vi "PID with autotuning.vi"(0 "gain scheduling variable":dbl format="%.2f", 4 "iteration":i32, 5 "autotuning parameters":T5={"Controller Type"=0, "# of cycles to avg"=3, "Relay amplitude"=2.0, "Control design  "=0, "Noise level"=0.1} {"Noise level" format="%.2f"; "Control design" items=["Normal", "Fast", "Slow"]; "Relay amplitude" format="%.2f"; "Controller Type" items=["PID", "PI", "P"]}, 6 "options":T3={"sp low"=0.0, "sp high"=100.0, "out low"=-100.0, "out high"=100.0, "hold (F)"=FALSE, "auto (T)"=TRUE, "pro. band (F)"=FALSE, "reverse acting (T)"=TRUE, "beta"=1.0, "linearity"=1.0, "dt (s)"=-1.0} {"dt (s)" format="%.2f"; "linearity" min=0.0 max=1.0 format="%.2f"; "sp low" format="%.2f"; "sp high" format="%.2f"; "out low" format="%.2f"; "out high" format="%.2f"; "beta" min=0.0 max=1.0 format="%.2f"}, 7 "autotune? (F)":bool, 8 "manual control":dbl(slide)=5.551115123125783e-15 scale=-100.0..100.0 scale format="%.1f", 9 "gain scheduling":T2={"gain schedule"=[100.0], "PID parameters"=[{"Kc"=4.851751673610237, "Ti (min)"=0.021111111111111112, "Td (min)"=0.005277777777777778}], "scheduling input"=0} {"scheduling input" items=["Setpoint", "Process variable", "Controller output", "Gain scheduling input"]; "PID parameters"."Td (min)" format="%.4f"; "PID parameters"."Ti (min)" format="%.4f"; "PID parameters"."Kc" format="%.4f"; "gain schedule" format="%.2f"}, 10 "process variable":dbl(slide)=29.68036460876465 scale=0.0..100.0 scale format="%.1f", 11 "setpoint":dbl(slide)=30.35714340209961 scale=0.0..100.0 scale format="%.1f") -> (1 "updated parameters":T2={"gain schedule"=[100.0], "PID parameters"=[{"Kc"=4.851751673610237, "Ti (min)"=0.021111111111111112, "Td (min)"=0.005277777777777778}], "scheduling input"=0} {"scheduling input" items=["Setpoint", "Process variable", "Controller output", "Gain scheduling input"]; "PID parameters"."Td (min)" format="%.4f"; "PID parameters"."Ti (min)" format="%.4f"; "PID parameters"."Kc" format="%.4f"; "gain schedule" format="%.2f"}, 2 "tuning completed?":bool, 3 "output":dbl(slide)=-0.9174311757087708 scale=-100.0..100.0 scale format="%.1f")   [LabVIEW 2020, in "NI_PID__autopid compat.lvlib"]
doc: "This VI can be used as a basic PID VI with gain scheduling. In addition, the VI has inputs used to specify and initiate a setpoint relay autotuning procedure. Passing a TRUE value to the autotune? input initiates the autotuning wizard.\n\nDescription of the PID algorithm:\n\nDerivative action is on the process variable only. Anti-reset windup and bumpless transfer are supported.\n\nThis VI should be called from inside a while loop with a fixed cycle time. If Cycle Time is less than or equal to zero, an internal timer with 1 millisecond resolution is used for calculations.\n\nThis VI is reentrant, so you can call it from multiple, independent higher-level VIs without interference.\n\nThe default variable ranges correspond to setpoint, process variable, and output expressed in percent. Reverse action (also called increase-decrease) is the \"normal\" controller mode where the output decreases if the process variable is higher than the setpoint.\n\nSwitching from auto to manual is bumpless; the initial value of the Manual Output control is subtracted out so that it is really a \"relative\" output control. Switching from manual to auto is also bumpless.\n\nSwitching to Hold causes the controller to ignore further changes in the process variable and suspends any integral action. Thus, the output stays constant at the last value."
uses:
  <vilib>/addons/control/pid/NI_PID__autopid compat.lvlib
  <vilib>/addons/control/pid/NI_PID__prctrl compat.lvlib
panel:
  in  "Dummy":T1 {"Td" format="%.2f"; "Ti" format="%.2f"; "Kc" format="%.2f"}
  in  "states":T4(ring)=enum."Start"
  # "SP & PV range:"
  # "Output range:"
  # "-1: default,using\nsystem clock"
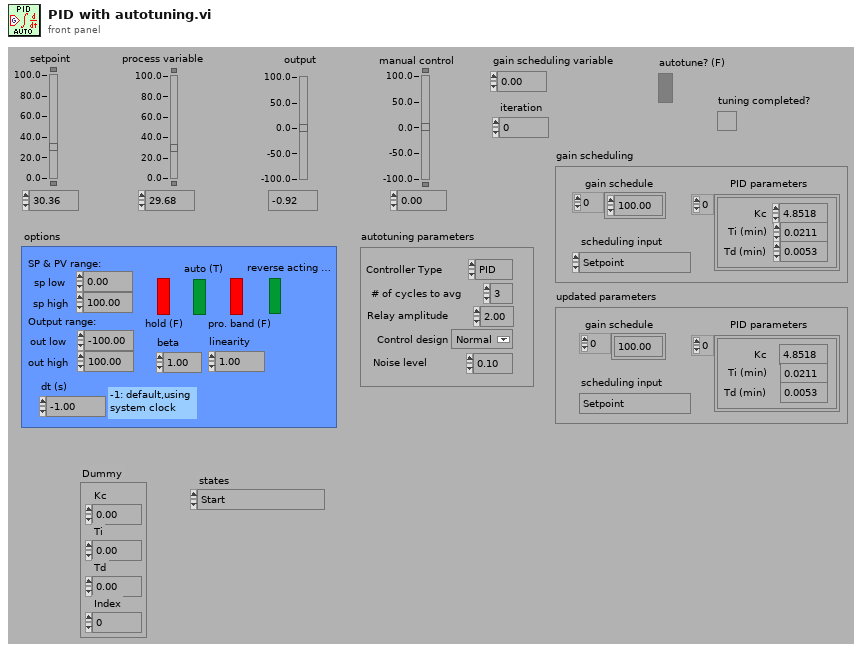
[diagram p1: front panel]
types:
  T1 = cluster{"Kc":dbl, "Ti":dbl, "Td":dbl, "Index":i32}
  T2 = cluster{"gain schedule":dbl[], "PID parameters":cluster{"Kc":dbl, "Ti (min)":dbl, "Td (min)":dbl}[], "scheduling input":u16}
  T3 = cluster{"sp low":dbl, "sp high":dbl, "out low":dbl, "out high":dbl, "hold (F)":bool, "auto (T)":bool, "pro. band (F)":bool, "reverse acting (T)":bool, "beta":dbl, "linearity":dbl, "dt (s)":dbl}
  T4 = enum16{"Normal", "Start", "Check params", "Check noise", "Start noise est.", "Re-estimate noise", "Begin autotune", "Autotuning", "New parameters", ""}
  T5 = cluster{"Controller Type":u16, "# of cycles to avg":i32, "Relay amplitude":dbl, "Control design  ":u16, "Noise level":dbl}
  T6 = cluster{"process variable":dbl, "setpoint relay":dbl, "output":dbl}
  T7 = cluster{"PB (%)":dbl, "Reset (min)":dbl, "Rate (min)":dbl, "Index":i32}
  T8 = cluster{"Kc":dbl, "Ti (min)":dbl, "Td (min)":dbl}[]
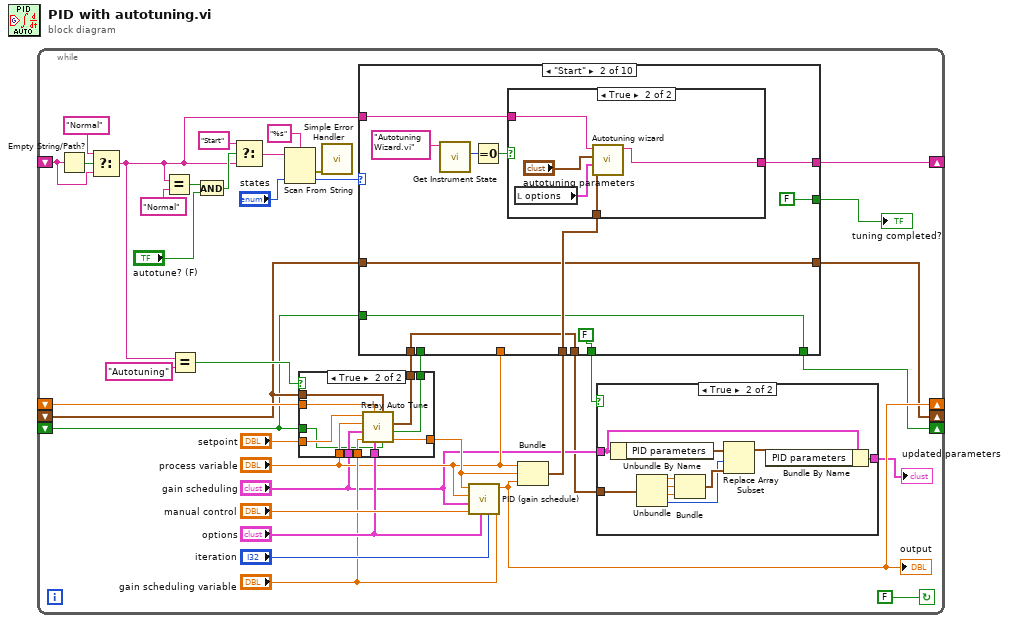
[diagram p0: block diagram]
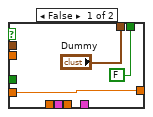
[diagram p3: hidden frame]
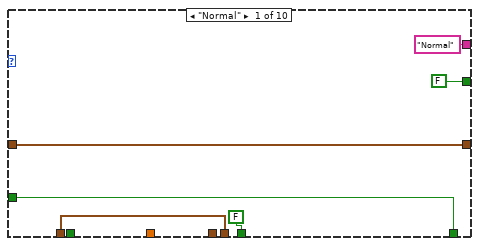
[diagram p4: hidden frame]
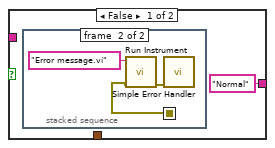
[diagram p5: hidden frame]
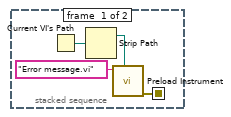
[diagram p6: hidden frame]
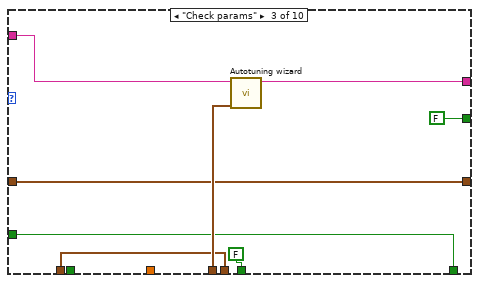
[diagram p7: hidden frame]
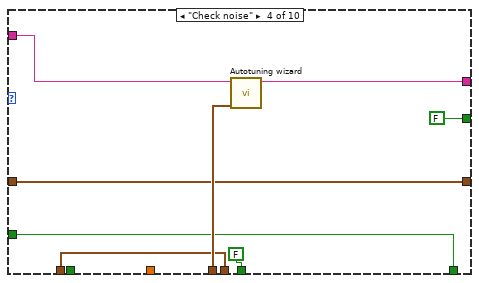
[diagram p8: hidden frame]
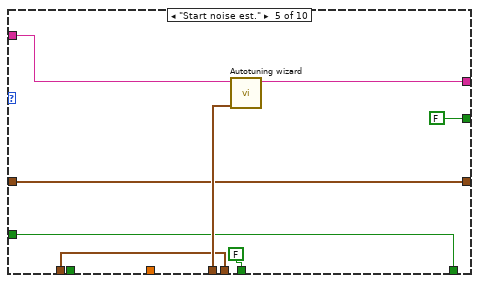
[diagram p9: hidden frame]
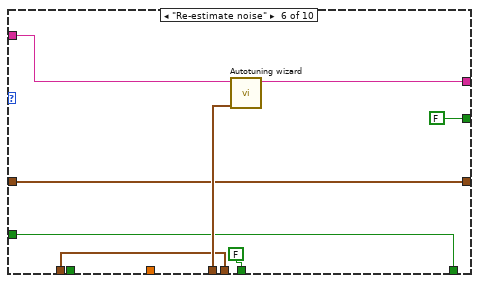
[diagram p10: hidden frame]
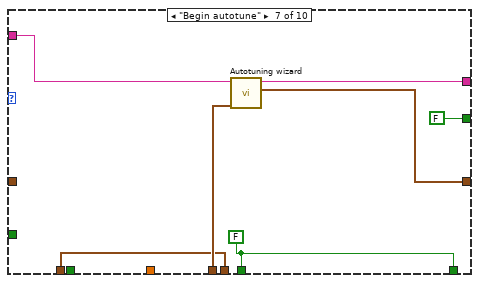
[diagram p11: hidden frame]
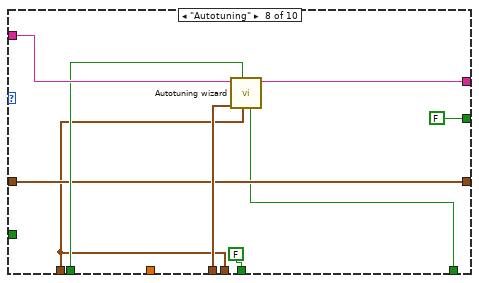
[diagram p12: hidden frame]
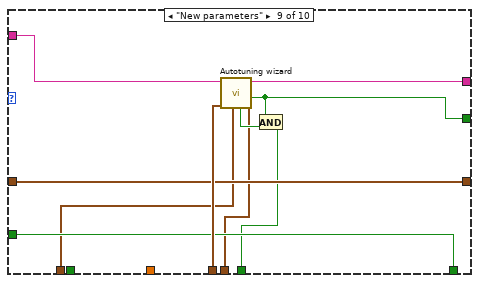
[diagram p13: hidden frame]
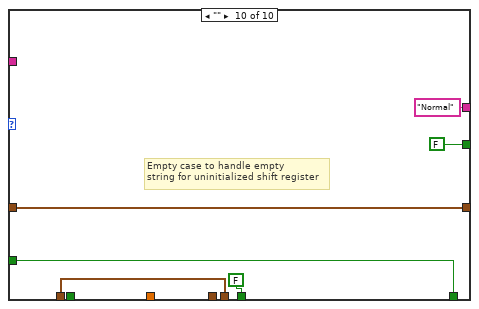
[diagram p14: hidden frame]
diagram:
  n1 = while {
    shift-left: _ -> [w12]
    shift-right: [w11] -> _
    shift-left: _ -> [w13]
    shift-right: [w14] -> _
    shift-left: _ -> [w27]
    shift-right: [w32] -> _
    shift-left: _ -> [w3]
    shift-right: [w38] -> _
    stop <- FALSE continue-if-true
    n2 = Empty String/Path?(string/path=w3) -> (empty?=w4:bool)
    n3 = Select(t="Normal", s=w4, f=w3) -> (s? t:f=w5:string)
    n4 = Equal?(x=w5, y="Normal") -> (x = y?=w6:bool)
    n5 = Equal?(x=w5, y="Autotuning") -> (x = y?=w23:bool)
    n6 = And(x=w6, y="autotune? (F)") -> (x .and. y?=w20:bool)
    n7 = Select(t="Start", s=w20, f=w5) -> (s? t:f=w19:string)
    n8 = Scan From String(format string="%s", input string=w19, default 1="states") -> (error out=w33:errorcluster, output 1=w36:T4)  [unwired: 2 in, 2 out]
    n9 = case shown="True" w23 {
      tunnel: [w53 w62] -> w28
      tunnel: "setpoint" -> [w53 w57]
      tunnel: w27 -> [_ w64]
      tunnel: ["Dummy" w63] -> w16
      tunnel: "options" -> [_ w61]
      tunnel: "gain scheduling variable" -> [_ w60]
      tunnel: "gain scheduling" -> [_ w59]
      tunnel: "process variable" -> [_ w58]
      tunnel: [FALSE ("tuning status") w56] -> w15
      tunnel: w13 -> [_ w55]
      tunnel: w12 -> [_ w54]
      frame False {
      }
      frame True {
        n10 = call <vilib>:"Relay Auto Tune.VI"("calculate"=w54, "autotuning parameters"=w55, "options"=w61, "Prev. control out"=w64, "Gain Scheduling Variable"=w60, "gain scheduling"=w59, "PV%"=w58, "setpoint (%)"=w57) -> ("setpoint relay"=w62:dbl, "tuning status"=w56:bool, "Tuned PID Parameters"=w63:T1)  [unwired: 1 out]
      }
    }
    n11 = call <vilib>:"Simple Error Handler.vi"("error in (no error)"=w33) -> ()  [unwired: 1 in, 8 out]
    n12 = call <vilib>:"PID (gain schedule).vi"("gain scheduling variable"="gain scheduling variable", "iteration"="iteration", "options"="options", "manual control"="manual control", "gain scheduling"="gain scheduling", "process variable"="process variable", "setpoint"=w28) -> ("output"=w32:dbl)  [unwired: 4 out]
    "output" <- w32
    n13 = Bundle("process variable"="process variable", "setpoint relay"=w28, "output"=w32) -> (w18:T6)  [unwired: 1 out]
    n14 = case shown="\"Start\"" w36 {
      tunnel: ["Normal" w80 w100 w108 w116 w124 w131 w140 w151 "Normal"] -> w38
      tunnel: [FALSE FALSE FALSE FALSE FALSE FALSE FALSE FALSE w145 FALSE] -> w39
      tunnel: w18 -> [_ w75 w99 w107 w115 w123 w130 w139 w150 _]
      tunnel: "process variable" -> [_ _ _ _ _ _ _ _ _ _]
      tunnel: w5 -> [_ w76 w101 w109 w117 w125 w132 w141 w152 _]
      tunnel: w16 -> [w66 w72 w96 w104 w112 w120 w128 w135 w144 w154]
      tunnel: w15 -> [_ _ _ _ _ _ _ w138 _ _]
      tunnel: [w68 w73 w98 w105 w113 w122 w129 w137 w149 w155] -> w14
      tunnel: w13 -> [w68 w73 w98 w105 w113 w122 _ w137 w149 w155]
      tunnel: [w67 w74 w97 w106 w114 w121 w127 w136 w148 w156] -> w11
      tunnel: w12 -> [w67 w74 w97 w106 w114 w121 _ _ w148 w156]
      tunnel: [FALSE FALSE FALSE FALSE FALSE FALSE w127 FALSE ("yes/no") w146 FALSE] -> w10
      tunnel: [w66 w72 w96 w104 w112 w120 w128 w135 w143 w154] -> w8
      frame "Normal" {
      }
      frame "Start" {
        n15 = call <vilib>:"Get Instrument State.vi"("VI name"="Autotuning Wizard.vi") -> ("window state"=w78:enum32{"Closed", "Open", "Open and Active"})  [unwired: 1 in, 9 out]
        n16 = Equal To 0?(x=w78) -> (x = 0?=w77:bool)
        n17 = case shown="True" w77 {
          tunnel: ["Normal" w92] -> w80
          tunnel: w76 -> [_ w93]
          tunnel: w75 -> [_ w91]
          frame False {
            n18 = stacked-sequence {
              seq-local: [w83 _] -> [_ w88]
              frame #0 {
                n19 = Current VI's Path() -> (path=w86:path)
                n20 = Strip Path(path=w86) -> (stripped path=w84:path)  [unwired: 1 out]
                n21 = call <vilib>:"Preload Instrument.vi"("VI path"=w84, "VI name"="Error message.vi") -> ("error out"=w83:errorcluster)  [unwired: 1 in, 8 out]
              }
              frame #1 {
                n22 = call <vilib>:"Run Instrument.vi"("error in (no error)"=w88, "VI name"="Error message.vi") -> ("error out"=w87:errorcluster)  [unwired: 9 out]
                n23 = call <vilib>:"Simple Error Handler.vi"("error in (no error)"=w87) -> ()  [unwired: 1 in, 8 out]
              }
            }
          }
          frame True {
            n24 = local read "options"() -> (w90:T3)
            n25 = call <vilib>:"Autotuning wizard.vi"("Control"=w91, "options"=w90, "autotuning parameters"="autotuning parameters", "current state"=w93) -> ("state"=w92:string)  [unwired: 2 in, 5 out]
          }
        }
      }
      frame "Check params" {
        n26 = call <vilib>:"Autotuning wizard.vi"("Control"=w99, "current state"=w101) -> ("state"=w100:string)  [unwired: 4 in, 5 out]
      }
      frame "Check noise" {
        n27 = call <vilib>:"Autotuning wizard.vi"("Control"=w107, "current state"=w109) -> ("state"=w108:string)  [unwired: 4 in, 5 out]
      }
      frame "Start noise est." {
        n28 = call <vilib>:"Autotuning wizard.vi"("Control"=w115, "current state"=w117) -> ("state"=w116:string)  [unwired: 4 in, 5 out]
      }
      frame "Re-estimate noise" {
        n29 = call <vilib>:"Autotuning wizard.vi"("Control"=w123, "current state"=w125) -> ("state"=w124:string)  [unwired: 4 in, 5 out]
      }
      frame "Begin autotune" {
        w127 = FALSE ("yes/no")
        n30 = call <vilib>:"Autotuning wizard.vi"("Control"=w130, "current state"=w132) -> ("autotuning parameters out"=w129:T5, "state"=w131:string)  [unwired: 4 in, 4 out]
      }
      frame "Autotuning" {
        n31 = call <vilib>:"Autotuning wizard.vi"("New PID Parameters input"=w135, "tuning completed?"=w138, "Control"=w139, "current state"=w141) -> ("state"=w140:string, "yes/no out"=w136:bool)  [unwired: 2 in, 4 out]
      }
      frame "New parameters" {
        n32 = call <vilib>:"Autotuning wizard.vi"("New PID Parameters input"=w144, "Control"=w150, "current state"=w152) -> ("New PID Parameters out"=w143:T7, "complete?"=w145:bool, "state"=w151:string, "yes/no out"=w147:bool)  [unwired: 3 in, 2 out]
        n33 = And(x=w145, y=w147) -> (x .and. y?=w146:bool)
      }
      frame "" {
        # "Empty case to handle empty\nstring for uninitialized shift register"
      }
    }
    "tuning completed?" <- w39
    n34 = case shown="True" w10 {
      tunnel: "gain scheduling" -> [w40 w42]
      tunnel: w8 -> [_ w43]
      tunnel: [w40 w41] -> w7
      frame False {
      }
      frame True {
        n35 = Unbundle By Name(w42) -> ("PID parameters"=w44:T8)
        n36 = Unbundle(w43) -> ("Kc"=w46:dbl, "Ti"=w47:dbl, "Td"=w48:dbl, "Index"=w45:i32)
        n37 = Bundle("Kc"=w46, "Ti"=w47, "Td"=w48) -> (w49:cluster{"Kc":dbl, "Ti":dbl, "Td":dbl})  [unwired: 1 out]
        n38 = Replace Array Subset(array=w44, new element=w49, index=w45) -> (w50:T8)
        n39 = Bundle By Name(cluster=w42, "PID parameters"=w50) -> (w41:T2)
      }
    }
    "updated parameters" <- w7
  }
